vi "Initialize System Actors.vi"(8 "error in (no error)":errorcluster, 10 "Root Actor In":refnum<class "Root Actor.lvclass">, 11 "System Modules Factory in":refnum<class "System Modules Factory.lvclass">) -> (0 "error out":errorcluster, 2 "Root Actor Out":refnum<class "Root Actor.lvclass">, 3 "System Modules Factory out":refnum<class "System Modules Factory.lvclass">)   [LabVIEW 2024, in "System Modules Factory.lvclass"]
uses:
  System Modules Factory.lvclass
  Actor/Root Actor/Root Actor.lvclass
  Messenger/Mail Strategy/Mail Strategy.lvclass
  System Modules Factory.lvclass/System Modules Factory.ctl
  General Parent Class/SEQ I64 Notifier/SEQ I64.lvclass
  Actor/System Actor/System Actor.lvclass/System Actor.ctl
  Actor/Root Actor/Root Actor.lvclass/Root Actor.ctl
  Actor/System Actor/Public Data/Write Self Messenger Location.vi
  Actor/System Actor/Public Data/Write Stop Notifier.vi
  Actor/System Actor/Public Data/Read ID.vi
  Actor/Root Actor/Protected Data/Accept VI Refs.vi
  Actor/Root Actor/Public Data/Write Modules Stop Notifier.vi
  Actor/System Actor/System Actor.lvclass
  General Parent Class/Enumeration Tree Queue Mailman/Enumeration Tree Queue Mailman.lvclass
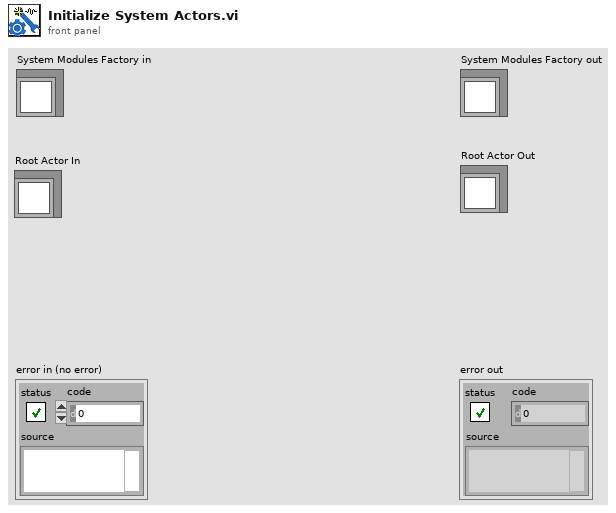
[diagram p1: front panel]
types:
  T1 = typedef "Config Parameters.ctl" = cluster{"Actors":refnum<class "System Actor.lvclass">[], "Rendevous Treads":i32[], "Actors Address":refnum<class "Mail Strategy.lvclass">[], "Root Actor Address":refnum<class "Mail Strategy.lvclass">}
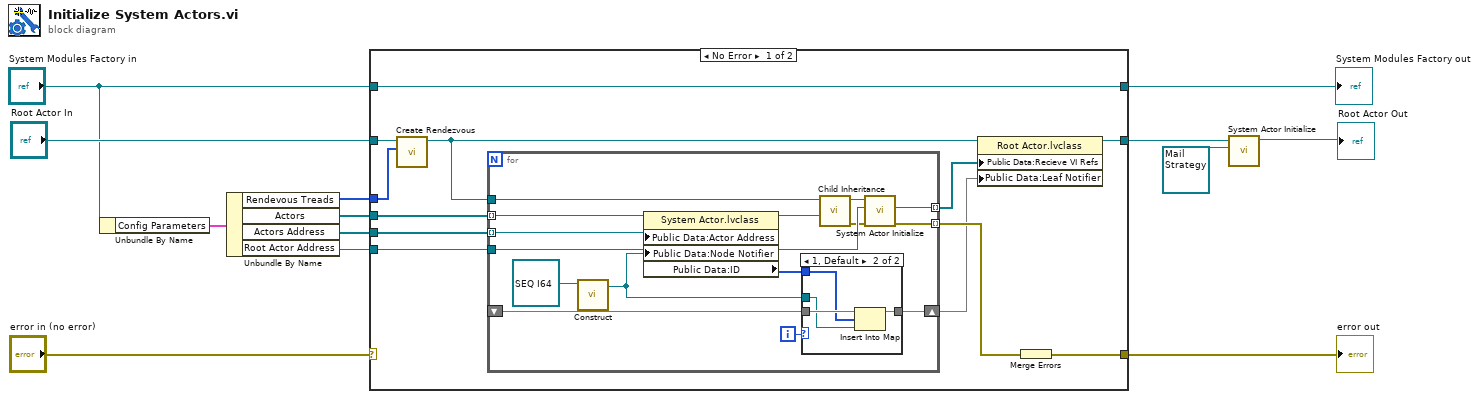
[diagram p0: block diagram]
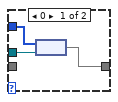
[diagram p2: hidden frame]
diagram:
  n1 = Unbundle By Name("System Modules Factory in") -> ("Config Parameters"=w1:T1)
  n2 = Unbundle By Name(w1) -> ("Rendevous Treads"=w10:i32[], "Actors"=w12:refnum<class "System Actor.lvclass">[], "Actors Address"=w11:refnum<class "Mail Strategy.lvclass">[], "Root Actor Address"=w9:refnum<class "Mail Strategy.lvclass">)
  n3 = case shown="No Error" "error in (no error)" {
    selector: "error in (no error)" -> [_ w50]
    tunnel: [w15 w50] -> w3
    tunnel: [w25 w49] -> w5
    tunnel: "System Modules Factory in" -> [w25 w49]
    tunnel: "Root Actor In" -> [w23 w48]
    tunnel: w12 -> [w24 _]
    tunnel: [w21 w48] -> w8
    tunnel: w11 -> [w20 _]
    tunnel: w10 -> [w19 _]
    tunnel: w9 -> [w18 _]
    frame No Error {
      n4 = call "Create Rendezvous.vi"("Treads"=w19, "Actor In"=w23) -> ("Actor Out"=w22:refnum<class "Root Actor.lvclass">)  [unwired: 8 in, 1 out]
      n5 = for {
        tunnel: w22 -> [w40]
        tunnel: w24 -> [w38] mode=indexing
        tunnel: [w39] -> w17 mode=indexing
        tunnel: w20 -> [w37] mode=indexing
        tunnel: w18 -> [w36]
        tunnel: [w32] -> w16 mode=indexing
        shift-right: [w29] -> w14
        shift-left: _ -> [w28]
        i -> [w31]
        n6 = call-dynamic "Construct.vi"("SEQ I64 in"=refnum<class "SEQ I64.lvclass"> refnum ("SEQ I64.lvclass")) -> ("SEQ I64 out"=w27:refnum<class "SEQ I64.lvclass">)  [unwired: 9 in, 1 out]
        n7 = property class="System Actor.lvclass"(reference=w38, "Public Data:Actor Address"=w37, "Public Data:Node Notifier"=w27) -> (reference out=w33:refnum<class "System Actor.lvclass">, "Public Data:ID"=w30:i64[])  [unwired: 1 in, 1 out]
        n8 = case shown="1, Default" w31 {
          tunnel: w30 -> [w42 w45]
          tunnel: w27 -> [w43 w44]
          tunnel: [w41 w46] -> w29
          tunnel: w28 -> [_ w47]
          frame 0 {
            n9 = node(w42, w43) -> (w41:map{i64[], refnum<class "SEQ I64.lvclass">})
          }
          frame 1, Default {
            n10 = Insert Into Map(map in=w47, key=w45, value=w44) -> (map out=w46:map{i64[], refnum<class "SEQ I64.lvclass">})  [unwired: 2 out]
          }
        }
        n11 = call "Child Inheritance.vi"("Child In"=w33, "Ancestor In"=w40) -> ("error out"=w34:errorcluster, "Child Out"=w35:refnum<class "System Actor.lvclass">)  [unwired: 8 in]
        n12 = call-dynamic "System Actor Initialize.vi"("error in (no error)"=w34, "Root Actor Address"=w36, "System Actor in"=w35) -> ("error out"=w32:errorcluster, "VI Refnum"=w39:refnum<vi>)  [unwired: 6 in, 1 out]
      }
      n13 = property class="Root Actor.lvclass"(reference=w22, "Public Data:Recieve VI Refs"=w17, "Public Data:Leaf Notifier"=w14) -> (reference out=w21:refnum<class "Root Actor.lvclass">)  [unwired: 1 in, 1 out]
      n14 = Merge Errors(w16) -> (w15:errorcluster)
    }
    frame Error {
    }
  }
  "error out" <- w3
  "System Modules Factory out" <- w5
  n15 = call-dynamic "System Actor Initialize.vi"("Root Actor Address"=refnum<class "Mail Strategy.lvclass"> refnum, "System Actor in"=w8) -> ("System Actor out"=→"Root Actor Out":refnum<class "Root Actor.lvclass">)  [unwired: 7 in, 2 out]
